vi "From Serial Form.vi"(6 "Serial Version":T1, 10 "Deserializer in":refnum<class "Deserializer.lvclass">, 11 "Test in":refnum<class "Test.lvclass">) -> (0 "error out":errorcluster, 2 "Deserializer out":refnum<class "Deserializer.lvclass">, 3 "Test out":refnum<class "Test.lvclass">)   [LabVIEW 2014, in "Test.lvclass"]
uses:
  Test.lvclass
  <vilib>/NI/AQ Character Lineator/Serializable/Serializable.lvclass
  <vilib>/NI/AQ Character Lineator/Serializable/Remove Data Value Reference of Serializable.vi
  <vilib>/NI/AQ Character Lineator/Serialization Common/Serial Version.ctl
  <vilib>/NI/AQ Character Lineator/Serialization Common/Serialization Common.lvlib
  <vilib>/NI/AQ Character Lineator/Deserializer/Deserializer.lvclass
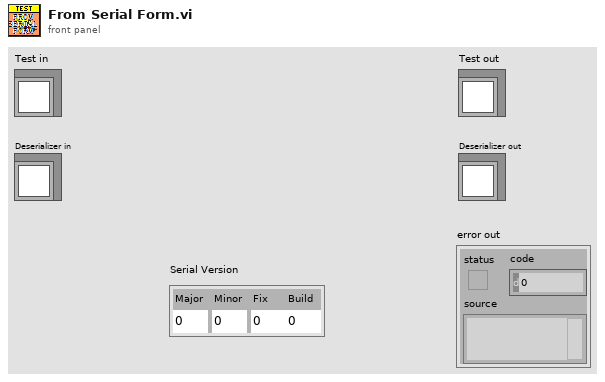
[diagram p1: front panel]
types:
  T1 = typedef "Serialization Common.lvlib/Serial Version.ctl" = cluster{"Major":u16, "Minor":u16, "Fix":u16, "Build":u16}
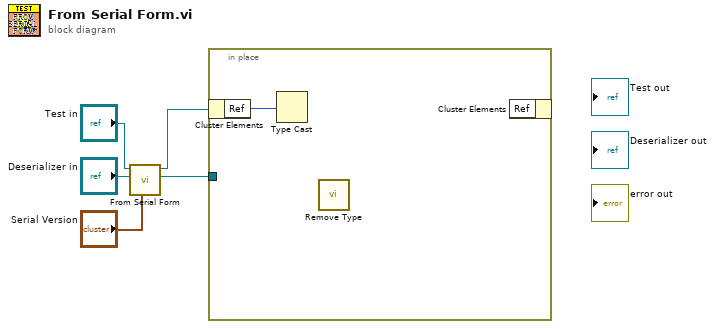
[diagram p0: block diagram]
diagram:
  n1 = call-parent "From Serial Form.vi"("Serial Version"="Serial Version", "Deserializer in"="Deserializer in", "Serializable in"="Test in") -> ("Deserializer out"=w2:refnum<class "Deserializer.lvclass">, "Serializable out"=w1:refnum<class "Test.lvclass">)  [unwired: 6 in, 1 out]
  n2 = in-place {
    in-place-border: w2 -> [_]
    n3 = in-place-cluster #1(w1) -> ("Ref"=w6:u32)
    n4 = Type Cast(x=w6) -> ()  [unwired: 1 in, 1 out]
    n5 = call-poly <vilib>:"Remove Type.vi"() -> ()  [unwired: 7 in, 5 out]
    n6 = in-place-cluster #1() -> ()  [unwired: 1 in, 1 out]
  }
